vi "Get Bitfile Object Ref.vi"(9 "scalar channel in":T2 {"Data Type" format="%.0x"}, 10 "bitfile object names":string[](array[string]), 11 "section children refs in":T1[](array[typedef]) format="%.0x") -> (1 "scalar channel out":T2 {"Data Type" format="%.0x"}, 2 "item ref out":T1=18446744073709551615 format="%.0x", 3 "section children refs out":T1[](array[typedef]) format="%.0x")   [LabVIEW 2018, in "FPGA Addon System Explorer.lvlib"]
uses:
  FPGA Addon System Explorer.lvlib
  Addon Shared/Types/Register Information.ctl
  Addon Shared/Types/Data Type.ctl
  <vilib>/NI Veristand/Custom Device API/Custom Device Item Ref.ctl
  <vilib>/NI Veristand/Custom Device API/Custom Device API.lvlib
  Addon Shared/FPGA Addon Shared.lvlib
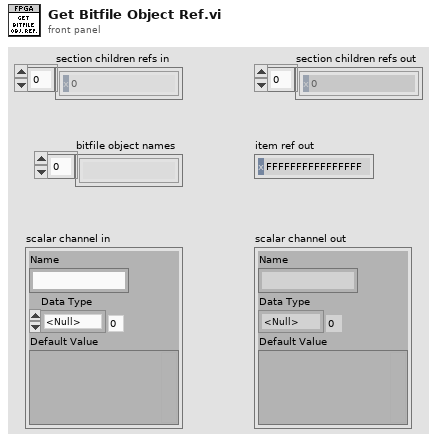
[diagram p1: front panel]
types:
  T1 = typedef "Custom Device API.lvlib/Custom Device Item Ref.ctl" = u64
  T2 = typedef "FPGA Addon Shared.lvlib/Register Information.ctl" = cluster{"Name":string, "Data Type":T3, "Default Value":variant}
  T3 = typedef "FPGA Addon Shared.lvlib/Data Type.ctl" = enum8{"<Null>", "I8", "I16", "I32", "I64", "U8", "U16", "U32", "U64", "SGL", "Boolean", "Analog PWM In Settings", "Analog PWM In", "Digital PWM In Settings", "Digital PWM In", "Digital PWM Out", "Sine Out", "FXP+/-24.5", "FXP+/-16.5", "FXP+/-32.8", "FXP+/-64.32", "FXP+/-16.7", "FXP+/-20.5", "FXP+/-27.5", "FXP+/-32.16", "FXP+16.3", "FXP+18.3", "Digital Static In", "Digital Static Out", "Digital Static In Settings", "Digital WSS Out", "Quad Encoder Settings", "Quad Encoder In", "Group"}
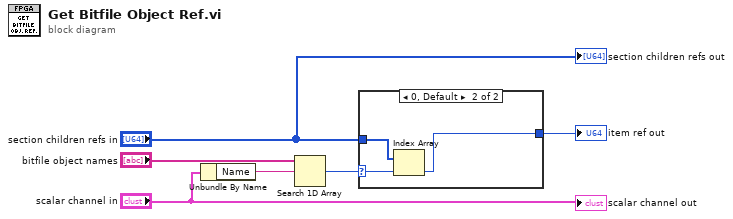
[diagram p0: block diagram]
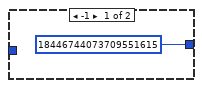
[diagram p2: hidden frame]
diagram:
  n1 = Unbundle By Name("scalar channel in") -> ("Name"=w4:string)
  n2 = Search 1D Array(1D array="bitfile object names", element=w4) -> (index of element=w2:i32)  [unwired: 1 in]
  n3 = case shown="0, Default" w2 {
    selector: w2 -> [_ w9]
    tunnel: "section children refs in" -> [_ w10]
    tunnel: [T1 18446744073709551615 ("Scalar Section ref") w8] -> w1
    frame -1 {
    }
    frame 0, Default {
      n4 = Index Array(array=w10, index=w9) -> (element=w8:T1)
    }
  }
  "item ref out" <- w1
  "scalar channel out" <- "scalar channel in"
  "section children refs out" <- "section children refs in"
